vi "ITX.Variant to String.vi"(8 "error in (no error)":errorcluster, 11 "Data (Variant)":variant) -> (0 "error out":errorcluster, 1 "Data":string, 2 "Size":string, 3 "Type":string)   [LabVIEW 2019, in "LV-Data.ITX.lvclass"]
uses:
  LV-Data.ITX.lvclass
  <vilib>/Utility/error.llb/Error Cluster From Error Code.vi
  <userlib>/_OpenG.lib/string/string.llb/Trim Whitespace (String)__ogtk.vi
  <vilib>/ErrorRing/Error Ring.xnode
  <vilib>/Utility/Data Type/NI_Data Type.lvlib
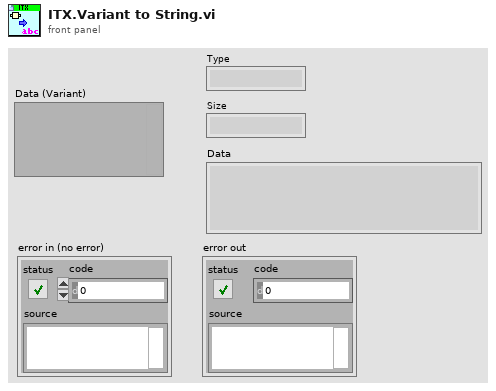
[diagram p1: front panel]
types:
  T1 = typedef "NI_Data Type.lvlib/Data Type.ctl" = enum8{"Invalid Type", "Void", "I8", "I16", "I32", "I64", "U8", "U16", "U32", "U64", "Single Float", "Double Float", "Extended Float", "Single Complex", "Double Complex", "Extended Complex", "Enum U8", "Enum U16", "Enum U32", "Enum U64", "Single Float With Unit", "Double Float With Unit", "Extended Float With Unit", "Single Complex with Unit", "Double Complex with Unit", "Extended Complex with Unit", "Boolean", "String", "Path", "Picture", "Tag", "Array", "Cluster", "Variant", "LV Variant", "Waveform", "Timestamp", "Digital Waveform", "Digital Data", "ExpressData", "Refnum", "External Data", "VI", "Poly VI", "LabVIEW Class Instance", "Fixed Point", "Set Collection", "Map Collection"}
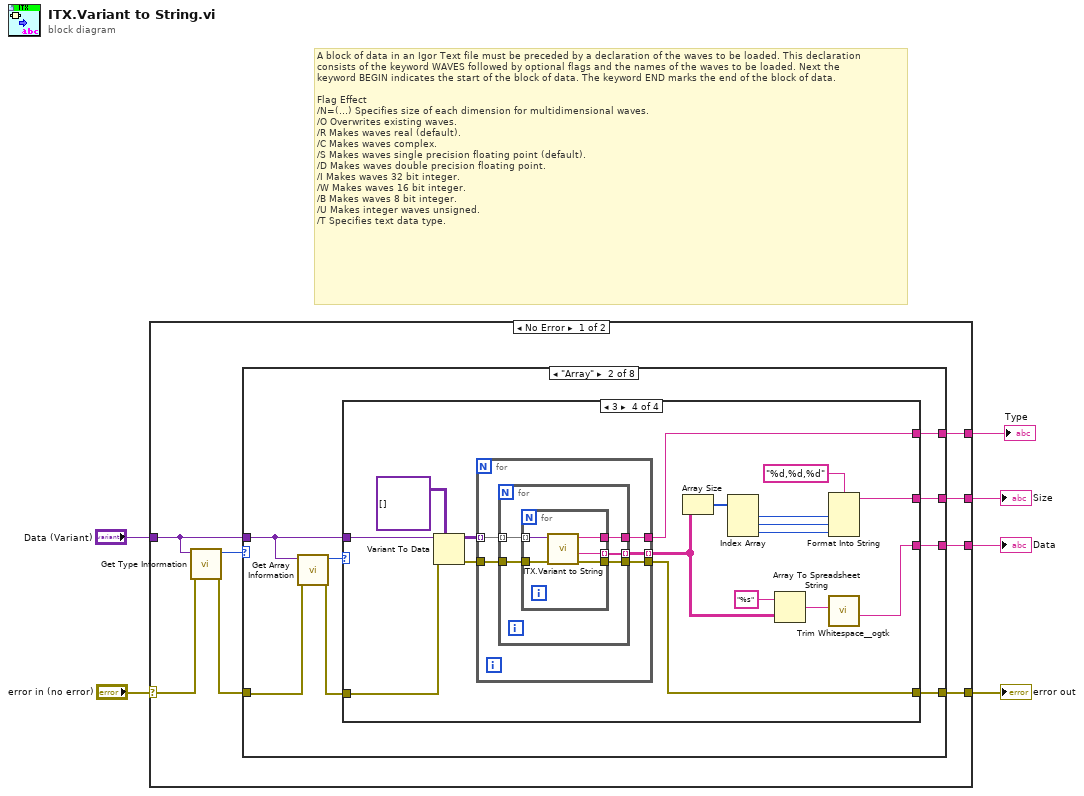
[diagram p0: block diagram]
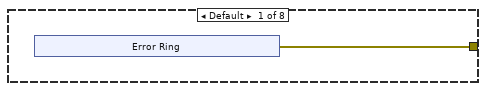
[diagram p2: hidden frame]
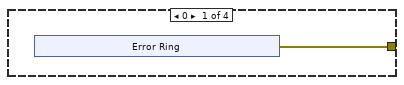
[diagram p3: hidden frame]
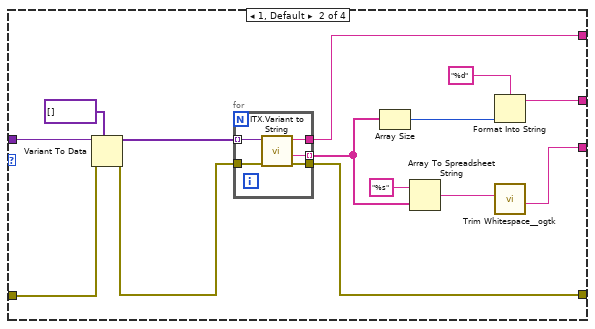
[diagram p4: hidden frame]
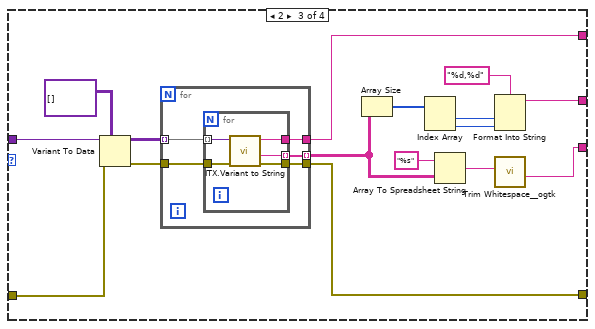
[diagram p5: hidden frame]
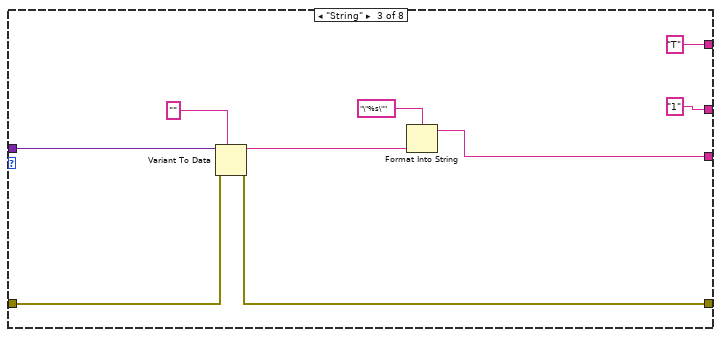
[diagram p6: hidden frame]
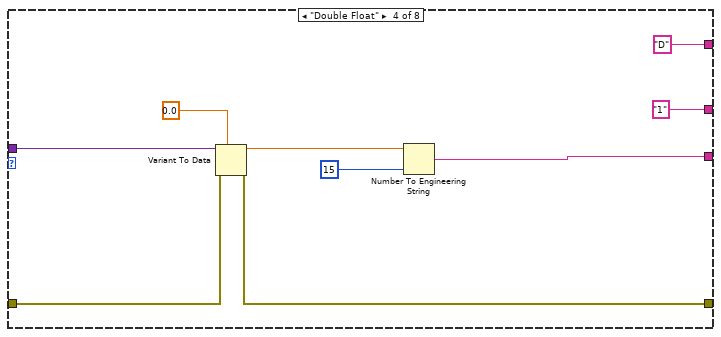
[diagram p7: hidden frame]
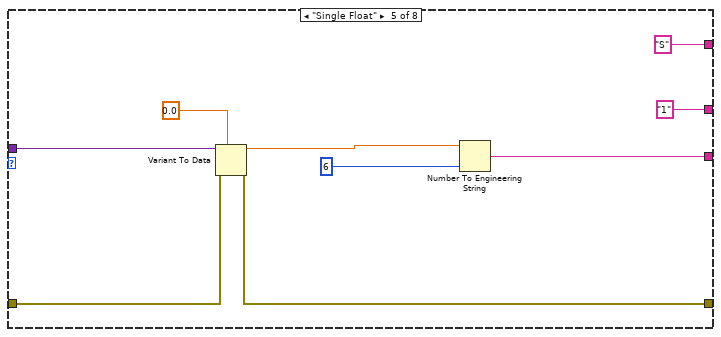
[diagram p8: hidden frame]
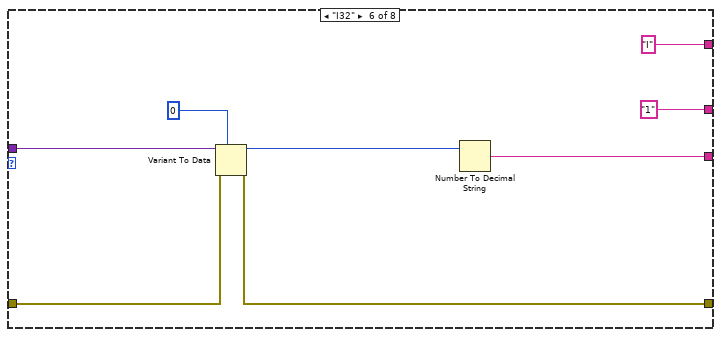
[diagram p9: hidden frame]
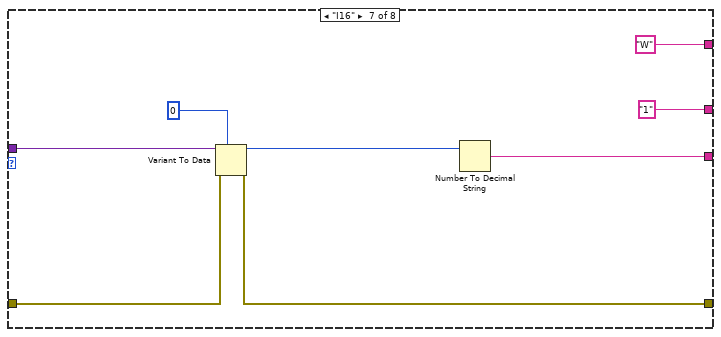
[diagram p10: hidden frame]
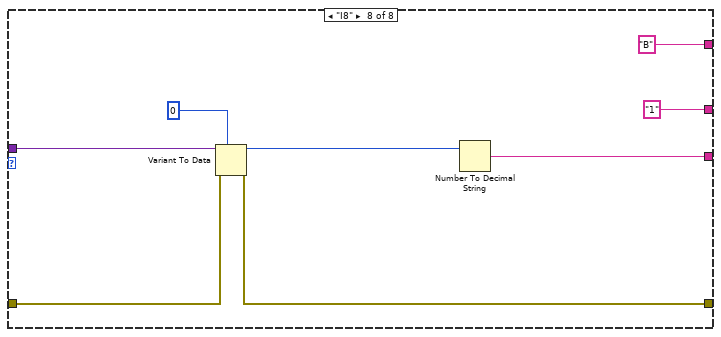
[diagram p11: hidden frame]
diagram:
  # "A block of data in an Igor Text file must be preceded by a declaration of the waves to be loaded. This declaration\nconsists of the keyword WAVES followed by optional flags and the names of the waves to be loaded. Next the\nkeyword BEGIN indicates the start of the block of data. The keyword END marks the end of the block of data.\n\nFlag Effect\n/N=(…) Specifies size of each dimension for multidimensional waves.\n/O Overwrites existing waves.\n/R Makes waves real (default).\n/C Makes waves complex.\n/S Makes waves single precision floating point (default).\n/D Makes waves double precision floating point.\n/I Makes waves 32 bit integer.\n/W Makes waves 16 bit integer.\n/B Makes waves 8 bit integer.\n/U Makes integer waves unsigned.\n/T Specifies text data type."
  n1 = case shown="No Error" "error in (no error)" {
    selector: "error in (no error)" -> [w8 w161]
    tunnel: [w14 w161] -> w6
    tunnel: "Data (Variant)" -> [w7 _]
    tunnel: [w13 _] -> w3
    tunnel: [w12 _] -> w2
    tunnel: [w11 _] -> w1
    frame No Error {
      n2 = call <vilib>:"Get Type Information.vi"("error in (no error)"=w8, "variant"=w7) -> ("error out"=w9:errorcluster, "type"=w10:T1)  [unwired: 5 in, 3 out]
      n3 = case shown="\"Array\"" w10 {
        tunnel: [w15 w27 w117 w125 w134 w142 w150 w158] -> w14
        tunnel: w7 -> [_ w22 w113 w127 w136 w144 w152 w160]
        tunnel: w9 -> [_ w26 w118 w126 w135 w143 w151 w159]
        tunnel: [_ w24 w111 w121 w130 w139 w147 w155] -> w13
        tunnel: [_ w23 "1" ("delimited string") "1" ("delimited string") "1" ("delimited string") "1" ("delimited string") "1" ("delimited string") "1" ("delimited string")] -> w12
        tunnel: [_ w21 "T" ("delimited string") "D" ("delimited string") "S" ("delimited string") "I" ("delimited string") "W" ("delimited string") "B" ("delimited string")] -> w11
        frame Default {
          n4 = xnode "Error Ring"() -> ("error out"=w15:errorcluster)
        }
        frame "Array" {
          n5 = call <vilib>:"Get Array Information.vi"("error in (no error)"=w26, "variant"=w22) -> ("error out"=w20:errorcluster, "number of dimensions"=w25:i32)  [unwired: 6 in, 2 out]
          n6 = case shown="3" w25 {
            tunnel: [w28 w40 w61 w88] -> w27
            tunnel: w22 -> [_ w44 w65 w92]
            tunnel: w20 -> [_ w45 w66 w93]
            tunnel: [_ w33 w56 w84] -> w24
            tunnel: [_ w37 w52 w82] -> w23
            tunnel: [_ w43 w64 w91] -> w21
            frame 0 {
              n7 = xnode "Error Ring"() -> ("error out"=w28:errorcluster)
            }
            frame 1, Default {
              n8 = Variant To Data(error in=w45, type=variant[] [], Variant=w44) -> (data=w42:variant[], error out=w41:errorcluster)
              n9 = for {
                tunnel: w42 -> [w51] mode=indexing
                tunnel: [w50] -> w34 mode=indexing
                tunnel: [w49] -> w43
                tunnel: w41 -> [w48]
                tunnel: [w47] -> w40
                n10 = call "ITX.Variant to String.vi"("error in (no error)"=w48, "Data (Variant)"=w51) -> ("error out"=w47:errorcluster, "Data"=w50:string, "Type"=w49:string)  [unwired: 6 in, 1 out]
              }
              n11 = Array Size(array=w34) -> (size(s)=w38:i32)
              n12 = Array To Spreadsheet String(array=w34, 3:"%s" ("format string")) -> (spreadsheet string=w35:string)  [unwired: 1 out]
              n13 = Format Into String(format string="%d", w38) -> (resulting string=w37:string)  [unwired: 2 in, 1 out]
              n14 = call-poly <userlib>:"Trim Whitespace__ogtk.vi"("String in"=w35) -> ("String out"=w33:string)  [unwired: 6 in]
            }
            frame 2 {
              n15 = Variant To Data(error in=w66, type=variant[][] [], Variant=w65) -> (data=w63:variant[][], error out=w62:errorcluster)
              n16 = for {
                tunnel: [w72] -> w64
                tunnel: w63 -> [w71] mode=indexing
                tunnel: [w70] -> w57 mode=indexing
                tunnel: w62 -> [w69]
                tunnel: [w68] -> w61
                n17 = for {
                  tunnel: w71 -> [w77] mode=indexing
                  tunnel: [w76] -> w70 mode=indexing
                  tunnel: [w75] -> w72
                  tunnel: w69 -> [w74]
                  tunnel: [w73] -> w68
                  n18 = call "ITX.Variant to String.vi"("error in (no error)"=w74, "Data (Variant)"=w77) -> ("error out"=w73:errorcluster, "Data"=w76:string, "Type"=w75:string)  [unwired: 6 in, 1 out]
                }
              }
              n19 = Array Size(array=w57) -> (size(s)=w60:i32[])
              n20 = Index Array(array=w60) -> (element #1=w54:i32, element #2=w53:i32)  [unwired: 2 in]
              n21 = Array To Spreadsheet String(array=w57, 3:"%s" ("format string")) -> (spreadsheet string=w58:string)  [unwired: 1 out]
              n22 = Format Into String(format string="%d,%d", w54, w53) -> (resulting string=w52:string)  [unwired: 2 in, 1 out]
              n23 = call-poly <userlib>:"Trim Whitespace__ogtk.vi"("String in"=w58) -> ("String out"=w56:string)  [unwired: 6 in]
            }
            frame 3 {
              n24 = Variant To Data(error in=w93, type=variant[][][] [], Variant=w92) -> (data=w90:variant[][][], error out=w89:errorcluster)
              n25 = for {
                tunnel: [w99] -> w91
                tunnel: w90 -> [w98] mode=indexing
                tunnel: [w95] -> w87 mode=indexing
                tunnel: w89 -> [w97]
                tunnel: [w96] -> w88
                n26 = for {
                  tunnel: [w104] -> w99
                  tunnel: w98 -> [w103] mode=indexing
                  tunnel: [w102] -> w95 mode=indexing
                  tunnel: w97 -> [w101]
                  tunnel: [w100] -> w96
                  n27 = for {
                    tunnel: w103 -> [w109] mode=indexing
                    tunnel: [w108] -> w102 mode=indexing
                    tunnel: [w107] -> w104
                    tunnel: w101 -> [w106]
                    tunnel: [w105] -> w100
                    n28 = call "ITX.Variant to String.vi"("error in (no error)"=w106, "Data (Variant)"=w109) -> ("error out"=w105:errorcluster, "Data"=w108:string, "Type"=w107:string)  [unwired: 6 in, 1 out]
                  }
                }
              }
              n29 = Array Size(array=w87) -> (size(s)=w81:i32[])
              n30 = Index Array(array=w81) -> (element #1=w80:i32, element #2=w79:i32, element #3=w78:i32)  [unwired: 3 in]
              n31 = Array To Spreadsheet String(array=w87, 3:"%s" ("format string")) -> (spreadsheet string=w85:string)  [unwired: 1 out]
              n32 = Format Into String(format string="%d,%d,%d", w80, w79, w78) -> (resulting string=w82:string)  [unwired: 2 in, 1 out]
              n33 = call-poly <userlib>:"Trim Whitespace__ogtk.vi"("String in"=w85) -> ("String out"=w84:string)  [unwired: 6 in]
            }
          }
        }
        frame "String" {
          n34 = Variant To Data(error in=w118, type="", Variant=w113) -> (data=w112:string, error out=w117:errorcluster)
          n35 = Format Into String(format string="\"%s\"", w112) -> (resulting string=w111:string)  [unwired: 2 in, 1 out]
        }
        frame "Double Float" {
          n36 = Variant To Data(error in=w126, type=0.0, Variant=w127) -> (data=w122:dbl, error out=w125:errorcluster)
          n37 = Number To Engineering String(2:i16 15 ("precision (6)"), 4:w122) -> (0:w121:string)  [unwired: 2 out]
        }
        frame "Single Float" {
          n38 = Variant To Data(error in=w135, type=sgl 0.0, Variant=w136) -> (data=w131:sgl, error out=w134:errorcluster)
          n39 = Number To Engineering String(2:i16 6 ("precision (6)"), 4:w131) -> (0:w130:string)  [unwired: 2 out]
        }
        frame "I32" {
          n40 = Variant To Data(error in=w143, type=0, Variant=w144) -> (data=w140:i32, error out=w142:errorcluster)
          n41 = Number To Decimal String(number=w140) -> (decimal integer string=w139:string)  [unwired: 1 in]
        }
        frame "I16" {
          n42 = Variant To Data(error in=w151, type=i16 0, Variant=w152) -> (data=w148:i16, error out=w150:errorcluster)
          n43 = Number To Decimal String(number=w148) -> (decimal integer string=w147:string)  [unwired: 1 in]
        }
        frame "I8" {
          n44 = Variant To Data(error in=w159, type=i16 0, Variant=w160) -> (data=w156:i16, error out=w158:errorcluster)
          n45 = Number To Decimal String(number=w156) -> (decimal integer string=w155:string)  [unwired: 1 in]
        }
      }
    }
    frame Error {
    }
  }
  "Data" <- w3
  "error out" <- w6
  "Size" <- w2
  "Type" <- w1
